vi "Test_sqlite3QueryVIM2DIntegerWorks_NoError.vi"(8 "error in (no error)":errorcluster, 11 "TestCase in":refnum<class "Test sqlite3.lvclass">) -> (0 "error out":errorcluster, 3 "TestCase out":refnum<class "Test sqlite3.lvclass">)   [LabVIEW 2020, in "Test sqlite3.lvclass"]
uses:
  Test sqlite3.lvclass
  Test sqlite3.lvclass/Test sqlite3.ctl
  <vilib>/addons/_JKI Toolkits/VI Tester/TestCase.llb/TestCase.lvclass
  45a547b6-e4c0-49d6-ab78-a1d3563bf804.vi
  externals/sqlite3/Source/sqlite3.lvclass
  externals/database-interface/IDatabase/IDatabase/IDatabase.lvclass
  C:/Program Files/National Instruments/LabVIEW 2020/vi.lib/addons/_JKI Toolkits/VI Tester/TestCase.llb/TestCase.lvclass
  C:/Users/Fred.Guo/Desktop/Database-configuration/externals/database-interface/Test/Test sqlite3/Test sqlite3.lvclass
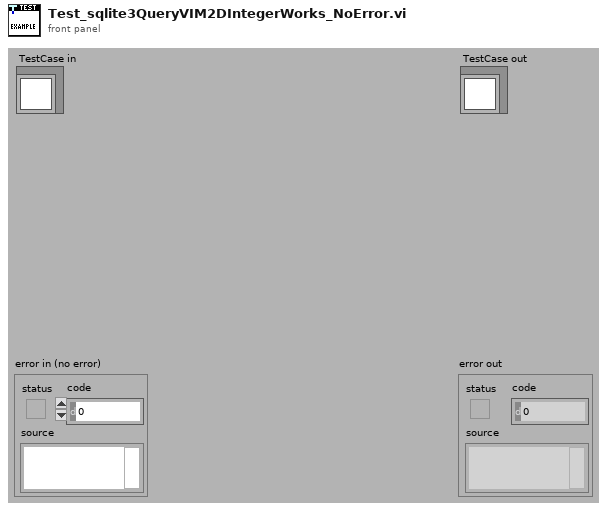
[diagram p1: front panel]
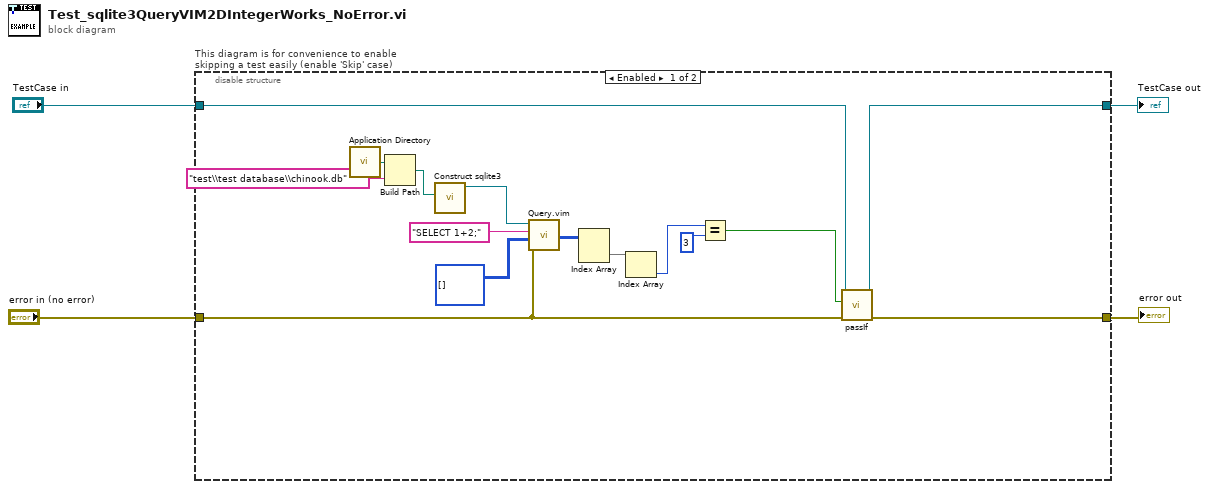
[diagram p0: block diagram]
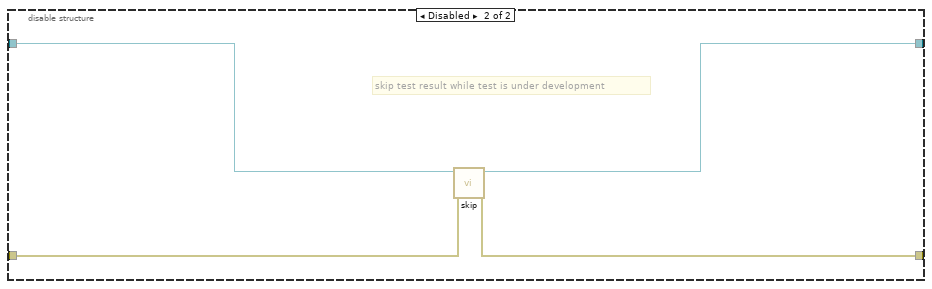
[diagram p2: hidden frame]
diagram:
  n1 = disable-structure "This diagram is for convenience to enable skipping a test easily (enable 'Skip' case)" shown="Enabled" {
    disable-tunnel: "TestCase in" -> [w17 w23]
    disable-tunnel: [w19 w21] -> w1
    disable-tunnel: [w18 w22] -> w3
    disable-tunnel: "error in (no error)" -> [w16 w20]
    frame Enabled {
      n2 = call <vilib>:"Application Directory.vi"() -> ("Application Directory"=w10:path)
      n3 = Build Path(base path=w10, name or relative path="test\\test database\\chinook.db") -> (appended path=w11:path)
      n4 = call "Construct sqlite3.vi"("DatabaseFilePath"=w11) -> ("sqlite3 out"=w6:refnum<class "sqlite3.lvclass">)  [unwired: 9 in, 1 out]
      n5 = call "Query.vim"("error in (no error)"=w16, "Type and Default"=i32[][] [] ("y"), "Query string"="SELECT 1+2;", "IDatabase in"=w6) -> ("Result"=w15:i32[][])  [unwired: 5 in, 2 out]
      n6 = Index Array(array=w15) -> (element=w14:i32[])  [unwired: 2 in]
      n7 = Index Array(array=w14) -> (element=w13:i32)  [unwired: 1 in]
      n8 = Equal?(x=w13, y=3) -> (x = y?=w12:bool)
      n9 = call-dynamic "passIf.vi"("error in (no error)"=w16, "pass"=w12, "TestCase in"=w17) -> ("error out"=w18:errorcluster, "TestCase out"=w19:refnum<class "Test sqlite3.lvclass">)  [unwired: 7 in]
    }
    frame Disabled {
      # "skip test result while test is under development"
      n10 = call <vilib>:"skip.vi"("error in (no error)"=w20, "TestCase in"=w23) -> ("error out"=w22:errorcluster, "TestCase out"=w21:refnum<class "Test sqlite3.lvclass">)  [unwired: 8 in]
    }
  }
  "error out" <- w3
  "TestCase out" <- w1
